vi "CfgFile Read Language File.vi"(8 "error in (no error)":errorcluster, 10 "Language Name":string, 11 "LF2R IDE in":refnum<class "LF2R IDE.lvclass">) -> (0 "error out":errorcluster, 1 "Exist?":bool, 2 "UI Descriptions":T1, 3 "LF2R IDE out":refnum<class "LF2R IDE.lvclass">)   [LabVIEW 2018, in "LF2R IDE.lvlib" / "LF2R IDE.lvclass"]
uses:
  LF2R IDE.lvclass
  Const UI Description Setting.ctl
  Const UI Desc Frame Title.ctl
  Const UI Desc Property.ctl
  Const UI Desc Frame Basic.ctl
  Const UI Desc Frame Skill.ctl
  Const UI Desc Frame bp.ctl
  Const UI Desc Frame w.ctl
  Const UI Desc Frame b.ctl
  Const UI Desc Frame i.ctl
  Const UI Desc Frame o.ctl
  Const UI Desc Frame c.ctl
  Const UI Desc Other.ctl
  Const UI Desc Menu.ctl
  136ff03b-022a-4f22-8316-e9f628dcce0b.vi
  <vilib>/JDP Science/JSONtext/JSON text to Variant.vi
  <vilib>/JDP Science/JSONtext/LVClass Serializer/JSONtext LVClass Serializer.lvclass
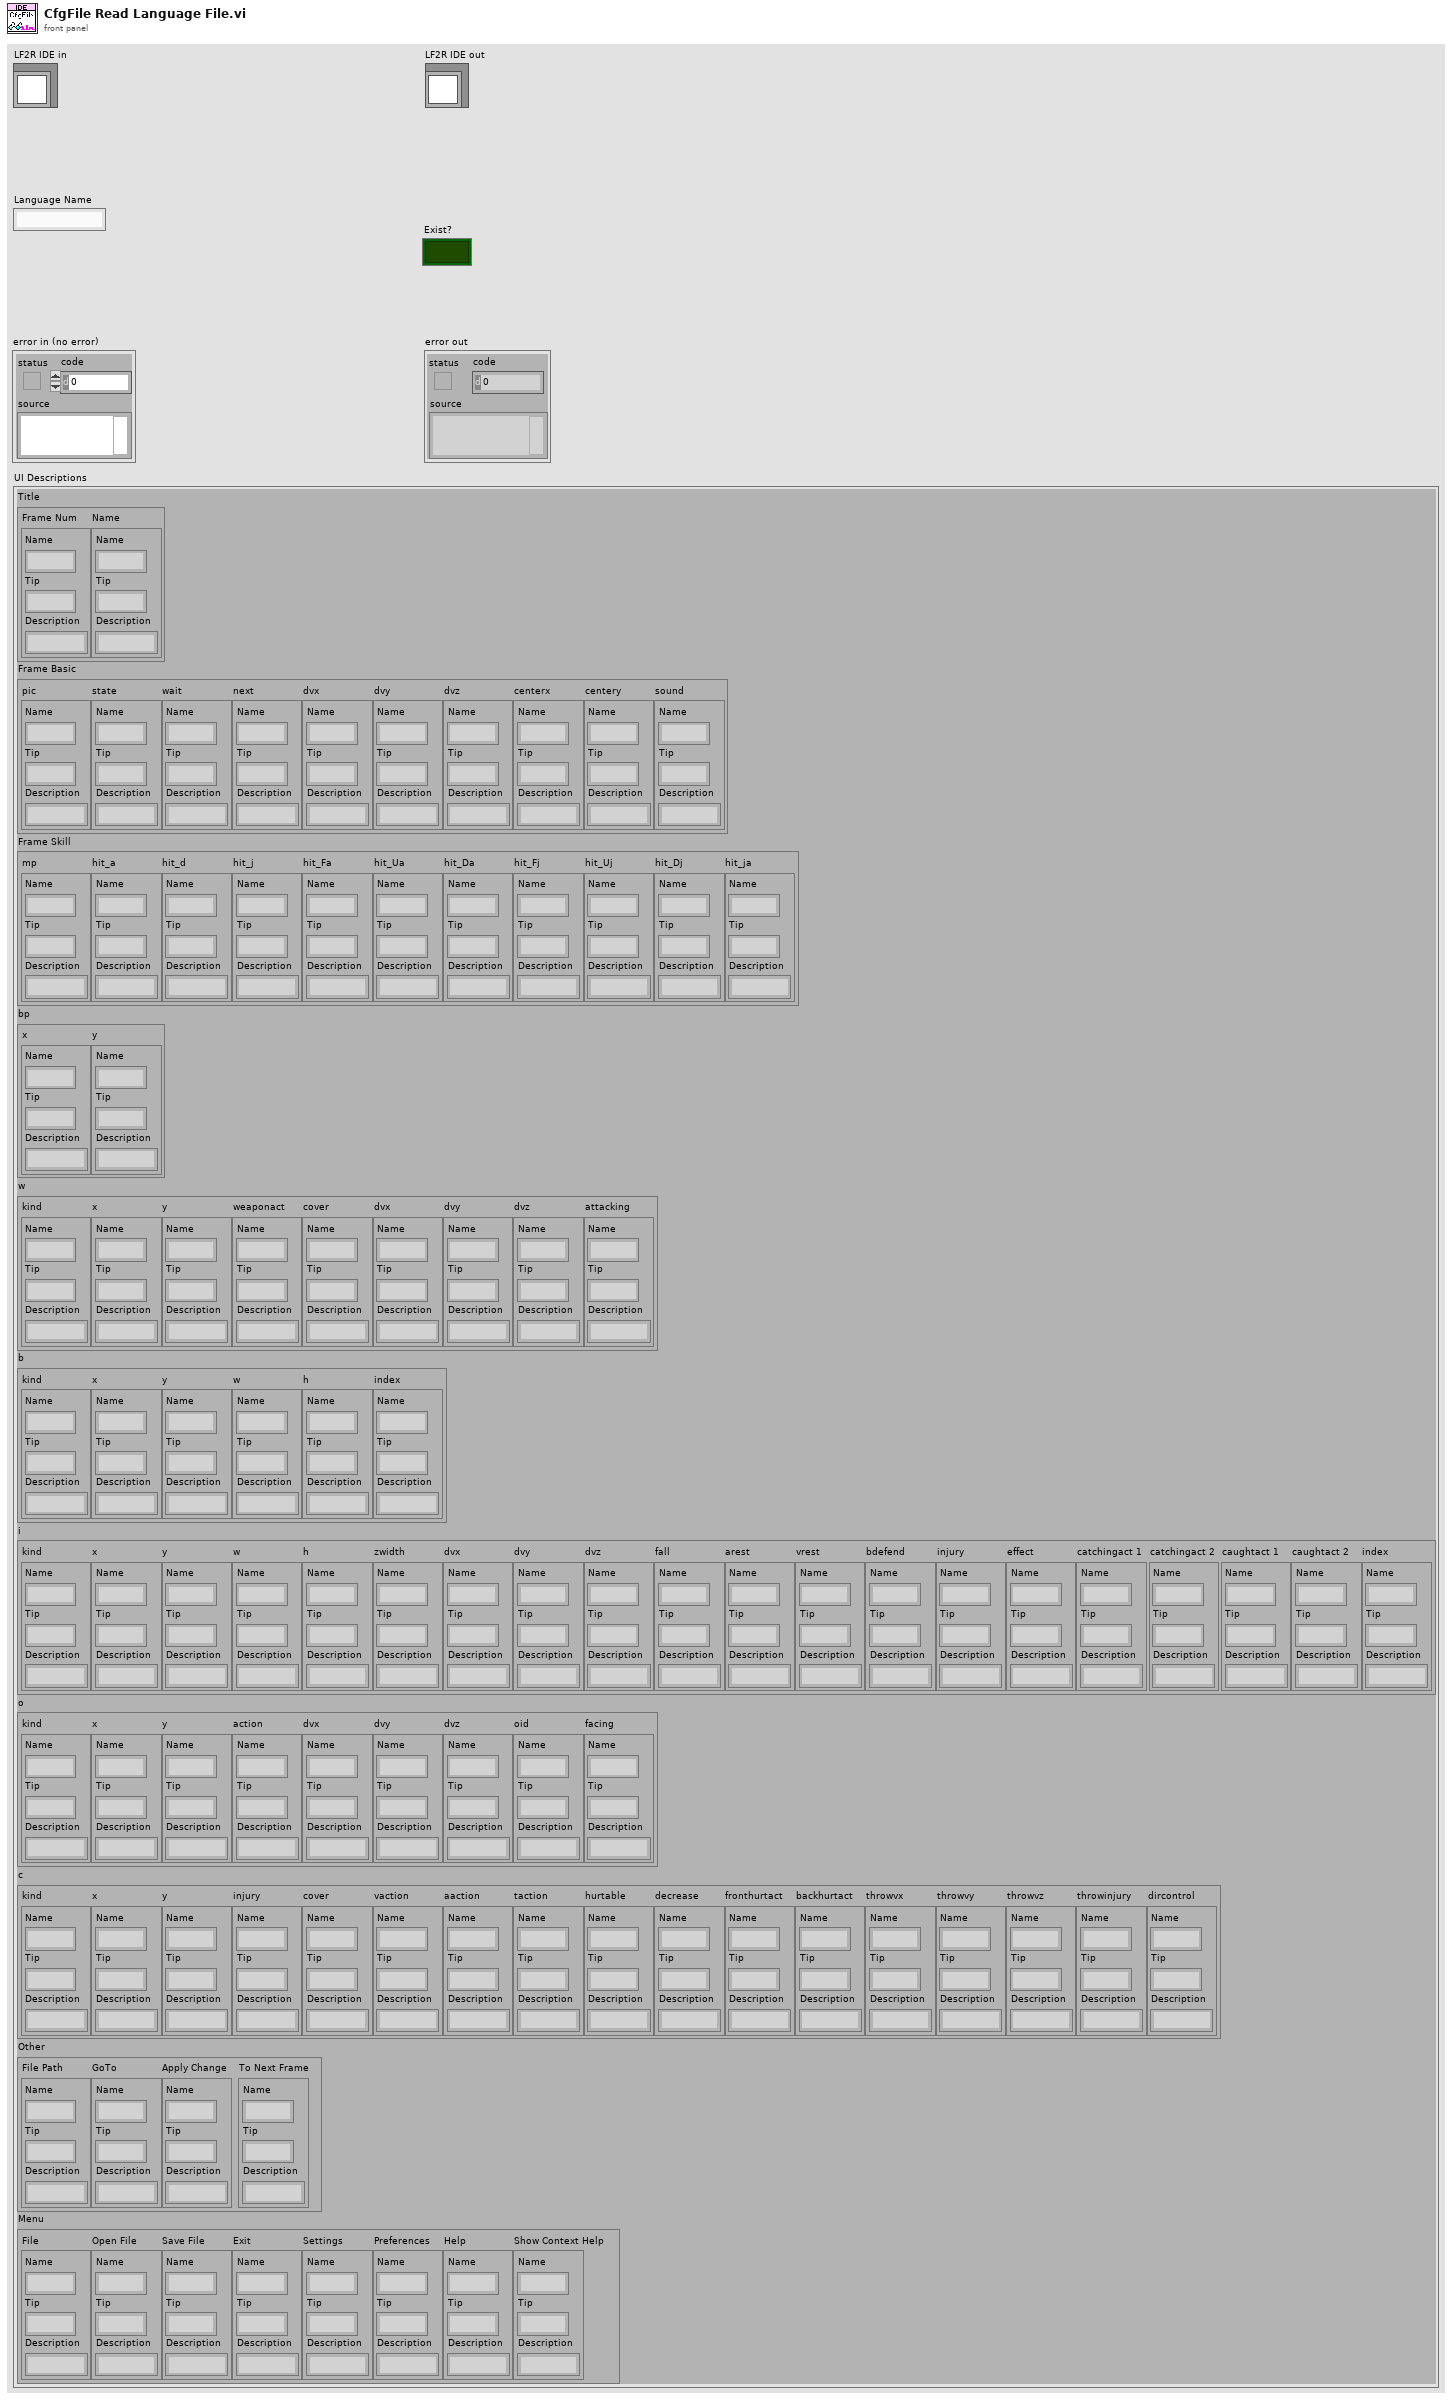
[diagram p1: front panel]
types:
  T1 = typedef "LF2R IDE.lvlib/LF2R IDE.lvclass/Const UI Description Setting.ctl" = cluster{"Title":T2, "Frame Basic":T4, "Frame Skill":T5, "bp":T6, "w":T7, "b":T8, "i":T9, "o":T10, "c":T11, "Other":T12, "Menu":T13}
  T2 = typedef "LF2R IDE.lvlib/LF2R IDE.lvclass/Const UI Desc Frame Title.ctl" = cluster{"Frame Num":T3, "Name":T3}
  T3 = typedef "LF2R IDE.lvlib/LF2R IDE.lvclass/Const UI Desc Property.ctl" = cluster{"Name":string, "Tip":string, "Description":string}
  T4 = typedef "LF2R IDE.lvlib/LF2R IDE.lvclass/Const UI Desc Frame Basic.ctl" = cluster{"pic":T3, "state":T3, "wait":T3, "next":T3, "dvx":T3, "dvy":T3, "dvz":T3, "centerx":T3, "centery":T3, "sound":T3}
  T5 = typedef "LF2R IDE.lvlib/LF2R IDE.lvclass/Const UI Desc Frame Skill.ctl" = cluster{"mp":T3, "hit_a":T3, "hit_d":T3, "hit_j":T3, "hit_Fa":T3, "hit_Ua":T3, "hit_Da":T3, "hit_Fj":T3, "hit_Uj":T3, "hit_Dj":T3, "hit_ja":T3}
  T6 = typedef "LF2R IDE.lvlib/LF2R IDE.lvclass/Const UI Desc Frame bp.ctl" = cluster{"x":T3, "y":T3}
  T7 = typedef "LF2R IDE.lvlib/LF2R IDE.lvclass/Const UI Desc Frame w.ctl" = cluster{"kind":T3, "x":T3, "y":T3, "weaponact":T3, "cover":T3, "dvx":T3, "dvy":T3, "dvz":T3, "attacking":T3}
  T8 = typedef "LF2R IDE.lvlib/LF2R IDE.lvclass/Const UI Desc Frame b.ctl" = cluster{"kind":T3, "x":T3, "y":T3, "w":T3, "h":T3, "index":T3}
  T9 = typedef "LF2R IDE.lvlib/LF2R IDE.lvclass/Const UI Desc Frame i.ctl" = cluster{"kind":T3, "x":T3, "y":T3, "w":T3, "h":T3, "zwidth":T3, "dvx":T3, "dvy":T3, "dvz":T3, "fall":T3, "arest":T3, "vrest":T3, "bdefend":T3, "injury":T3, "effect":T3, "catchingact 1":T3, "catchingact 2":T3, "caughtact 1":T3, "caughtact 2":T3, "index":T3}
  T10 = typedef "LF2R IDE.lvlib/LF2R IDE.lvclass/Const UI Desc Frame o.ctl" = cluster{"kind":T3, "x":T3, "y":T3, "action":T3, "dvx":T3, "dvy":T3, "dvz":T3, "oid":T3, "facing":T3}
  T11 = typedef "LF2R IDE.lvlib/LF2R IDE.lvclass/Const UI Desc Frame c.ctl" = cluster{"kind":T3, "x":T3, "y":T3, "injury":T3, "cover":T3, "vaction":T3, "aaction":T3, "taction":T3, "hurtable":T3, "decrease":T3, "fronthurtact":T3, "backhurtact":T3, "throwvx":T3, "throwvy":T3, "throwvz":T3, "throwinjury":T3, "dircontrol":T3}
  T12 = typedef "LF2R IDE.lvlib/LF2R IDE.lvclass/Const UI Desc Other.ctl" = cluster{"File Path":T3, "GoTo":T3, "Apply Change":T3, "To Next Frame":T3}
  T13 = typedef "LF2R IDE.lvlib/LF2R IDE.lvclass/Const UI Desc Menu.ctl" = cluster{"File":T3, "Open File":T3, "Save File":T3, "Exit":T3, "Settings":T3, "Preferences":T3, "Help":T3, "Show Context Help":T3}
  T14 = enum16{"open", "replace", "create", "open or create", "replace or create", "replace or create with confirmation"}
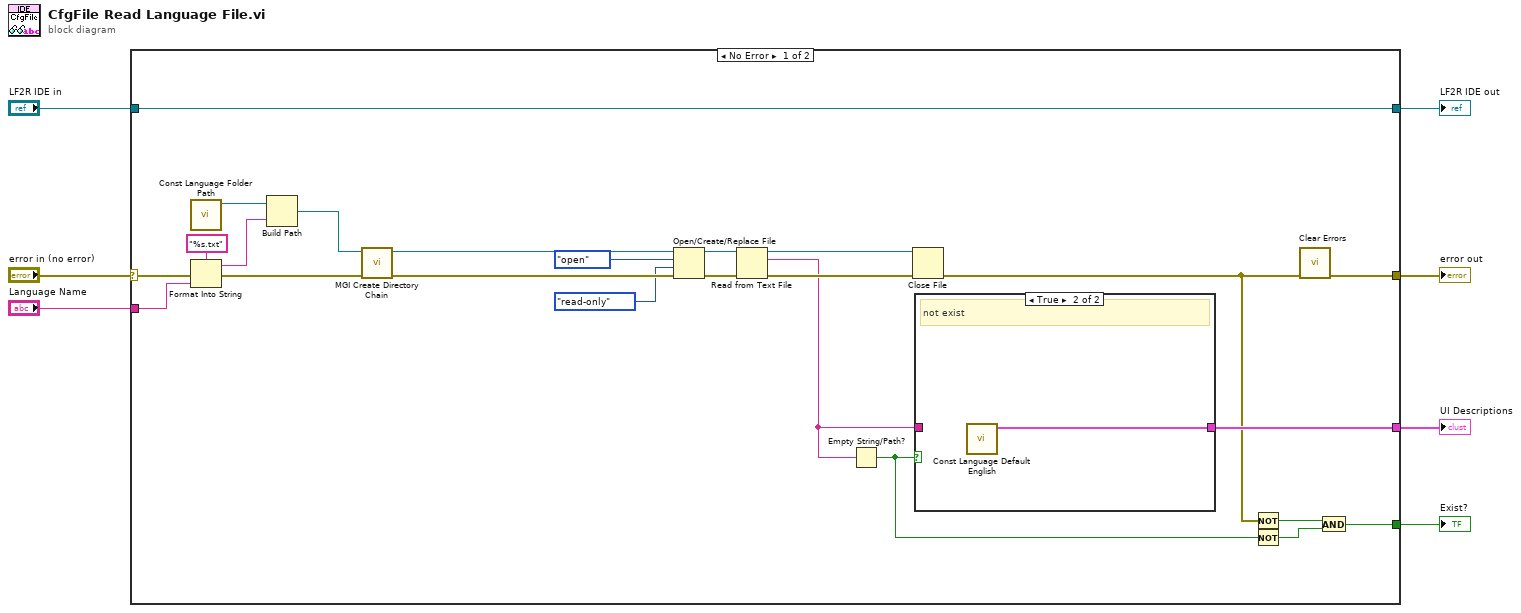
[diagram p0: block diagram]
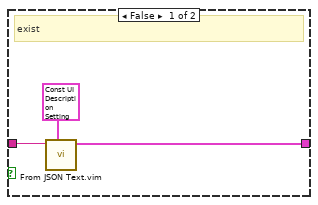
[diagram p2: hidden frame]
diagram:
  n1 = case shown="No Error" "error in (no error)" {
    selector: "error in (no error)" -> [w10 w37]
    tunnel: [w20 w37] -> w6
    tunnel: [w25 w36] -> w4
    tunnel: "LF2R IDE in" -> [w25 w36]
    tunnel: [w21 _] -> w1
    tunnel: [w17 _] -> w3
    tunnel: "Language Name" -> [w13 _]
    frame No Error {
      n2 = call "Const Language Folder Path.vi"() -> ("Language Folder Path"=w14:path)  [unwired: 11 in]
      n3 = Format Into String(format string="%s.txt", error in=w10, w13) -> (resulting string=w11:string, error out=w9:errorcluster)  [unwired: 1 in]
      n4 = Build Path(base path=w14, name or relative path=w11) -> (appended path=w8:path)
      n5 = call <userlib>:"MGI Create Directory Chain.vi"("Error In"=w9, "Path"=w8) -> ("Error Out"=w30:errorcluster, "Duplicate Path"=w31:path)  [unwired: 8 in]
      n6 = Open/Create/Replace File(file path (use dialog)=w31, error in=w30, operation (0:open)=T14."open", access (0:read/write)=enum16{"read/write", "read-only", "write-only"}."read-only") -> (refnum out=w29:refnum<file>, error out=w28:errorcluster)  [unwired: 2 in, 1 out]
      n7 = Read from Text File(file (use dialog)=w29, error in=w28) -> (refnum out=w27:refnum<file>, text=w22:string, error out=w24:errorcluster)  [unwired: 2 in, 1 out]
      n8 = Empty String/Path?(string/path=w22) -> (empty?=w19:bool)
      n9 = Close File(refnum=w27, error in=w24) -> (error out=w15:errorcluster)  [unwired: 1 out]
      n10 = case shown="True" w19 {
        tunnel: [w33 w35] -> w21
        tunnel: w22 -> [w34 _]
        frame False {
          # "exist"
          n11 = call "From JSON Text.vim"("Data Type and Default Value"=T1 {"Title"={"Frame Num"={"Name"="", "Tip"="", "Description"=""}, "Name"={"Name"="", "Tip"="", "Description"=""}}, "Frame Basic"={"pic"={"Name"="", "Tip"="", "Description"=""}, "state"={"Name"="", "Tip"="", "Description"=""}, "wait"={"Name"="", "Tip"="", "Description"=""}, "next"={"Name"="", "Tip"="", "Description"=""}, "dvx"={"Name"="", "Tip"="", "Description"=""}, "dvy"={"Name"="", "Tip"="", "Description"=""}, "dvz"={"Name"="", "Tip"="", "Description"=""}, "centerx"={"Name"="", "Tip"="", "Description"=""}, "centery"={"Name"="", "Tip"="", "Description"=""}, "sound"={"Name"="", "Tip"="", "Description"=""}}, "Frame Skill"={"mp"={"Name"="", "Tip"="", "Description"=""}, "hit_a"={"Name"="", "Tip"="", "Description"=""}, "hit_d"={"Name"="", "Tip"="", "Description"=""}, "hit_j"={"Name"="", "Tip"="", "Description"=""}, "hit_Fa"={"Name"="", "Tip"="", "Description"=""}, "hit_Ua"={"Name"="", "Tip"="", "Description"=""}, "hit_Da"={"Name"="", "Tip"="", "Description"=""}, "hit_Fj"={"Name"="", "Tip"="", "Description"=""}, "hit_Uj"={"Name"="", "Tip"="", "Description"=""}, "hit_Dj"={"Name"="", "Tip"="", "Description"=""}, "hit_ja"={"Name"="", "Tip"="", "Description"=""}}, "bp"={"x"={"Name"="", "Tip"="", "Description"=""}, "y"={"Name"="", "Tip"="", "Description"=""}}, "w"={"kind"={"Name"="", "Tip"="", "Description"=""}, "x"={"Name"="", "Tip"="", "Description"=""}, "y"={"Name"="", "Tip"="", "Description"=""}, "weaponact"={"Name"="", "Tip"="", "Description"=""}, "cover"={"Name"="", "Tip"="", "Description"=""}, "dvx"={"Name"="", "Tip"="", "Description"=""}, "dvy"={"Name"="", "Tip"="", "Description"=""}, "dvz"={"Name"="", "Tip"="", "Description"=""}, "attacking"={"Name"="", "Tip"="", "Description"=""}}, "b"={"kind"={"Name"="", "Tip"="", "Description"=""}, "x"={"Name"="", "Tip"="", "Description"=""}, "y"={"Name"="", "Tip"="", "Description"=""}, "w"={"Name"="", "Tip"="", "Description"=""}, "h"={"Name"="", "Tip"="", "Description"=""}, "index"={"Name"="", "Tip"="", "Description"=""}}, "i"={"kind"={"Name"="", "Tip"="", "Description"=""}, "x"={"Name"="", "Tip"="", "Description"=""}, "y"={"Name"="", "Tip"="", "Description"=""}, "w"={"Name"="", "Tip"="", "Description"=""}, "h"={"Name"="", "Tip"="", "Description"=""}, "zwidth"={"Name"="", "Tip"="", "Description"=""}, "dvx"={"Name"="", "Tip"="", "Description"=""}, "dvy"={"Name"="", "Tip"="", "Description"=""}, "dvz"={"Name"="", "Tip"="", "Description"=""}, "fall"={"Name"="", "Tip"="", "Description"=""}, "arest"={"Name"="", "Tip"="", "Description"=""}, "vrest"={"Name"="", "Tip"="", "Description"=""}, "bdefend"={"Name"="", "Tip"="", "Description"=""}, "injury"={"Name"="", "Tip"="", "Description"=""}, "effect"={"Name"="", "Tip"="", "Description"=""}, "catchingact 1"={"Name"="", "Tip"="", "Description"=""}, "catchingact 2"={"Name"="", "Tip"="", "Description"=""}, "caughtact 1"={"Name"="", "Tip"="", "Description"=""}, "caughtact 2"={"Name"="", "Tip"="", "Description"=""}, "index"={"Name"="", "Tip"="", "Description"=""}}, "o"={"kind"={"Name"="", "Tip"="", "Description"=""}, "x"={"Name"="", "Tip"="", "Description"=""}, "y"={"Name"="", "Tip"="", "Description"=""}, "action"={"Name"="", "Tip"="", "Description"=""}, "dvx"={"Name"="", "Tip"="", "Description"=""}, "dvy"={"Name"="", "Tip"="", "Description"=""}, "dvz"={"Name"="", "Tip"="", "Description"=""}, "oid"={"Name"="", "Tip"="", "Description"=""}, "facing"={"Name"="", "Tip"="", "Description"=""}}, "c"={"kind"={"Name"="", "Tip"="", "Description"=""}, "x"={"Name"="", "Tip"="", "Description"=""}, "y"={"Name"="", "Tip"="", "Description"=""}, "injury"={"Name"="", "Tip"="", "Description"=""}, "cover"={"Name"="", "Tip"="", "Description"=""}, "vaction"={"Name"="", "Tip"="", "Description"=""}, "aaction"={"Name"="", "Tip"="", "Description"=""}, "taction"={"Name"="", "Tip"="", "Description"=""}, "hurtable"={"Name"="", "Tip"="", "Description"=""}, "decrease"={"Name"="", "Tip"="", "Description"=""}, "fronthurtact"={"Name"="", "Tip"="", "Description"=""}, "backhurtact"={"Name"="", "Tip"="", "Description"=""}, "throwvx"={"Name"="", "Tip"="", "Description"=""}, "throwvy"={"Name"="", "Tip"="", "Description"=""}, "throwvz"={"Name"="", "Tip"="", "Description"=""}, "throwinjury"={"Name"="", "Tip"="", "Description"=""}, "dircontrol"={"Name"="", "Tip"="", "Description"=""}}, "Other"={"File Path"={"Name"="", "Tip"="", "Description"=""}, "GoTo"={"Name"="", "Tip"="", "Description"=""}, "Apply Change"={"Name"="", "Tip"="", "Description"=""}, "To Next Frame"={"Name"="", "Tip"="", "Description"=""}}, "Menu"={"File"={"Name"="", "Tip"="", "Description"=""}, "Open File"={"Name"="", "Tip"="", "Description"=""}, "Save File"={"Name"="", "Tip"="", "Description"=""}, "Exit"={"Name"="", "Tip"="", "Description"=""}, "Settings"={"Name"="", "Tip"="", "Description"=""}, "Preferences"={"Name"="", "Tip"="", "Description"=""}, "Help"={"Name"="", "Tip"="", "Description"=""}, "Show Context Help"={"Name"="", "Tip"="", "Description"=""}}} ("UI Descriptions"), "JSON"=w34) -> ("Data out"=w33:T1)  [unwired: 8 in, 1 out]
        }
        frame True {
          # "not exist"
          n12 = call "Const Language Default English.vi"() -> ("UI Descriptions"=w35:T1)  [unwired: 11 in]
        }
      }
      n13 = Not(x=w15) -> (.not. x?=w18:bool)
      n14 = Not(x=w19) -> (.not. x?=w16:bool)
      n15 = call <vilib>:"Clear Errors.vi"("error in (no error)"=w15) -> ("error out"=w20:errorcluster)  [unwired: 5 in, 1 out]
      n16 = And(x=w18, y=w16) -> (x .and. y?=w17:bool)
    }
    frame Error {
    }
  }
  "error out" <- w6
  "LF2R IDE out" <- w4
  "Exist?" <- w3
  "UI Descriptions" <- w1
